vi "UHR-Fleezers Control (host) -Leonardo 04-2018 V1.vi"(0 "Tab Control":T5(tab)=enum."Trap Control (RF)") -> ()   [LabVIEW 2013] (continued)
  n85 = xnode "Read/Write Control"("FPGA VI Reference In"=w151, "error in"=w171, "ai count"="AI Count (ticks)", "Interlace ON/OFF"=w137, "Number Interlace Cycles"=w136, "Set 1"=w16, "Set 2"=w15, "Set 3"=w14, "FB On/Off Set 1"=w258, "FB On/Off Set 2"=w257, "Interlace Off Parameters"=w135, "FB Setpoint Set 1"=w249, "FB Setpoint Set 2"=w248, "FB Gains"="PID gains", "FB output range"=cluster{"output high":i16, "output low":i16} {"output high"=3000, "output low"=0} ("FB output range 1"), "Cycles per step"=w234, "Scan BD"=w246, "Number of scans"=w230, "Scan steps"=w235, "Scan freq.  increment"=w236, "AO1 (Y)"=w218, "AO2 (X)"=w217, "Scan freq.  increment (MCL)"=w211, "Scan steps (MCL)"=w210, "Cycles per step (MCL)"=w209, "Number of scans (MCL)"=w208, "MCL count"=w134, "Cont. Scan (MCL)"=w207, "MCL Scan Axis"=w201, "1D or 2D Scan?"=w154, "N of AI1 Int Acq Sets"=w191, "BD 1 Delay (ticks)"="Freq switch delay", "Amp switch delay"="Amp switch delay", "Swap F1 and F2"="Swap F1 and F2", "APD Acq Rate Count"=w159, "APD to FIFO"=FALSE, "APD Gate Operating Mode"="APD Gate", "APD Gate ON Count"="APD Gate ON Count", "APD Gate OFF Count"="APD Gate OFF Count", "Invert APD Gate"="Invert APD Gate", "DIO count 1 (ticks)"="DIO count 1 (ticks)", "DIO count 2 (ticks)"="DIO count 2 (ticks)", "DIO count 3 (ticks)"="DIO count 3 (ticks)", "APD 1 AO scale factor"="APD 1 AO Mult.", "APD 2 AO scale factor"="APD 2 AO Mult.", "Diff FB Measurement?"=w21, "Dynamic Force FB (Ronen)"=w20, "Negate Diff?"=w19, "Next trap write delay (ticks)"="Next trap write delay (ticks)", "Phase offset method"="Phase offset method", "Phase Trap 1"="Phase increment trap 1", "RF phase reset before cycles"="RF phase reset before cycles", "Phase Trap 2"="Phase increment trap 2") -> ("FPGA VI Reference Out"=w129:T20, "error out"=w131:errorcluster)  [unwired: 1 in]
  n86 = local read "Green Laser ON/Interlacing"() -> (w132:bool)
  n87 = local read "Green laser mode"() -> (w133:enum32{"Laser ON", "Laser OFF", "Interlace"})
  n88 = local read "GI Frequency, OFF count"() -> (w125:u32)
  n89 = local read "GI Frequency, ON count"() -> (w124:u32)
  n90 = Multiply(x="Current When FB OFF (%)", y=655.35) -> (x*y=w115:dbl)
  n91 = local read "Green FB Count"() -> (w123:u32)
  n92 = Multiply(x="Green FB Setpoint (mV)", y=3.2767) -> (x*y=w112:dbl)
  n93 = To Unsigned Word Integer(number=w115) -> (unsigned 16bit integer=w113:u16)
  n94 = local read "Invert GI"() -> (w127:bool)
  n95 = To Word Integer(number=w112) -> (16bit integer=w110:i16)
  n96 = case shown="True" w132 {
    tunnel: w133 -> [_ w293]
    tunnel: [enum32{"Laser ON", "Laser OFF", "Interlace"}."Laser OFF" ("Green laser mode") w293] -> w126
    frame False {
    }
    frame True {
    }
  }
  n97 = local read "Trap Pos. AI1 X Pre-scale"() -> (w81:u16)
  n98 = local read "Trap Pos FB Monitor\nT1 or T2"() -> (w88:bool)
  n99 = local read "Trap Pos FB Int Count"() -> (w78:u16)
  n100 = local read "Trap Pos FB Negate Action"() -> (w87:bool)
  n101 = local read "Trap Pos. FB Offset Factor"() -> (w86:i64)
  n102 = local read "Trap Pos. FB Mult Factor"() -> (w85:i64)
  n103 = local read "Trap Pos. FB Gains"() -> (w83:T11)
  n104 = local read "Trap Pos. FB Range"() -> (w84:T12)
  n105 = xnode "Read/Write Control"("FPGA VI Reference In"=w129, "error in"=w131, "Green interlace ON count 2"=w124, "Green interlace OFF count 2"=w125, "Invert GI 2"=w127, "Operating Mode 2"=w126, "Green FB Gains"="Green FB Gains", "Green FB Setpoint"=w110, "Green FB On/Off"="Green FB On/Off", "Current Out"=w113, "Green int current ON count adj"="Green int current ON count adj", "Green FB Count"=w123, "Operating Mode"=w126, "Green interlace OFF count"=w125, "Green interlace ON count"=w124, "Invert GI"=w127, "Trap Pos FB Monitor T1 or T2"=w88, "Trap Pos FB Negate Action"=w87, "Trap Pos. FB Offset Factor"=w86, "Trap Pos. FB Mult Factor"=w85, "Trap pos. FB Range"=w84, "Trap Pos. FB Gains"=w83, "Force feedback"=FALSE, "AI1 X Scale"=w81, "Trap Pos to FIFO"=TRUE, "Trap Pos FB Int Count"=w78) -> ("FPGA VI Reference Out"=w128:T20, "error out"=w130:errorcluster)
  n106 = xnode "Invoke Method"("FPGA VI Reference In"=w128, "error in"=w130, "Requested Depth"="Trap AI FIFO Depth") -> ("FPGA VI Reference Out"=w91:T20, "error out"=w90:errorcluster)  [unwired: 1 out]
  n107 = xnode "Invoke Method"("FPGA VI Reference In"=w91, "error in"=w90, "Requested Depth"="Trap Position FIFO Depth") -> ("FPGA VI Reference Out"=w4:T20, "error out"=w2:errorcluster)  [unwired: 1 out]
  n108 = xnode "Invoke Method"("FPGA VI Reference In"=w4, "error in"=w2, "Requested Depth"="APD FIFO Depth (requires restart)") -> ("FPGA VI Reference Out"=w3:T20, "error out"=w1:errorcluster)  [unwired: 1 out]
  n109 = flat-sequence {
    tunnel: w152 -> [w298]
    tunnel: [w298] -> w151
    tunnel: [w294] -> w37
    tunnel: [w297] -> w150
    tunnel: [w296] -> w148
    tunnel: [w295] -> w149
    frame #0 {
      w295 = T16 {"Minimum"=60.0, "Maximum"=90.0, "Increment"=1.0} ("Min Max Inc")
      w296 = T16 {"Minimum"=0.0, "Maximum"=75.0, "Increment"=1.0} ("Data Entry Limits")
      w294 = T16 {"Minimum"=60.0, "Maximum"=90.0, "Increment"=1.0} ("Min Max Inc")
      w297 = T16 {"Minimum"=0.0, "Maximum"=75.0, "Increment"=1.0} ("Data Entry Limits")
      n110 = property on="BD 2 Frequency 1 (MHz)" class="DigNum (strict)"("Data Range"=w295) -> ()  [unwired: 2 in, 2 out]
      n111 = property on="BD 2 Frequency 3 (MHz)" class="DigNum (strict)"("Data Range"=w295) -> ()  [unwired: 2 in, 2 out]
      n112 = property on="BD 2 Frequency 2 (MHz)" class="DigNum (strict)"("Data Range"=w295) -> ()  [unwired: 2 in, 2 out]
      n113 = property on="BD 1 Frequency 1 (MHz)" class="DigNum (strict)"("Data Range"=w294) -> ()  [unwired: 2 in, 2 out]
      n114 = property on="BD 1 Frequency 2 (MHz)" class="DigNum (strict)"("Data Range"=w294) -> ()  [unwired: 2 in, 2 out]
      n115 = property on="BD 1 Frequency 3 (MHz)" class="DigNum (strict)"("Data Range"=w294) -> ()  [unwired: 2 in, 2 out]
      n116 = property on="BD 2 Amplitude 1 (%)" class="DigNum (strict)"("Data Range"=w296) -> ()  [unwired: 2 in, 2 out]
      n117 = property on="BD 2 Amplitude 2 (%)" class="DigNum (strict)"("Data Range"=w296) -> ()  [unwired: 2 in, 2 out]
      n118 = property on="BD 2 Amplitude 3 (%)" class="DigNum (strict)"("Data Range"=w296) -> ()  [unwired: 2 in, 2 out]
      n119 = property on="BD 1 Amplitude 3 (%)" class="DigNum (strict)"("Data Range"=w297) -> ()  [unwired: 2 in, 2 out]
      n120 = property on="BD 1 Amplitude 2 (%)" class="DigNum (strict)"("Data Range"=w297) -> ()  [unwired: 2 in, 2 out]
      n121 = property on="BD 1 Amplitude 1 (%)" class="DigNum (strict)"("Data Range"=w297) -> ()  [unwired: 2 in, 2 out]
      "X RF Frequency Limits (MHz)" <- w294
      "X RF Amplitude Limits (%)" <- w297
      "Y RF Amplitude Limits (%)" <- w296
      "Y RF Frequency Limits (MHz)" <- w295
    }
  }
  n122 = xnode "Invoke Method"("FPGA VI Reference In"=w3, "error in"=w1) -> ("FPGA VI Reference Out"=w57:T20, "error out"=w56:errorcluster)  [unwired: 1 in]
  n123 = flat-sequence "Initial FPGA Loop Relative Phase Adjustment" {
    tunnel: "Initial Phase Adjustment (APD 2 Gate)" -> [w300]
    tunnel: "Initial Phase Adjustment (GI) 2" -> [w301]
    tunnel: "Initial Phase Adj. (MCL)" -> [w302]
    tunnel: w56 -> [w303]
    tunnel: w57 -> [w304]
    tunnel: "Initial Phase Adjustment (GI)" -> [w305]
    tunnel: "Initial Phase Adjustment (AI1)" -> [w306]
    tunnel: [w306] -> w66
    tunnel: [w305] -> w65
    tunnel: [w304] -> w64
    tunnel: [w303] -> w63
    tunnel: [w302] -> w62
    tunnel: [w301] -> w61
    tunnel: [w300] -> w60
    tunnel: [w318] -> w177
    tunnel: [w312] -> w175
    tunnel: "Initial Phase Adjustment (APD Acq)" -> [w311]
    tunnel: "Initial Phase Adjustment (APD 1 Gate)" -> [w310]
    tunnel: "Initial Phase Adjustment (Green FB)" -> [w309]
    tunnel: w66 -> [w317]
    tunnel: w65 -> [w316]
    tunnel: w64 -> [w315]
    tunnel: w63 -> [w314]
    tunnel: w62 -> [w313]
    tunnel: w61 -> [w308]
    tunnel: w60 -> [w307]
    tunnel: w177 -> [w320]
    tunnel: [w321] -> w176
    tunnel: w175 -> [w321]
    tunnel: [w320] -> w174
    tunnel: w176 -> [w324]
    tunnel: w174 -> [w323]
    tunnel: [w326] -> w173
    tunnel: [w325] -> w172
    tunnel: [w328] -> w55
    tunnel: [w329] -> w58
    tunnel: w173 -> [w329]
    tunnel: w172 -> [w328]
    frame #0 {
      n124 = Wait (ms)(milliseconds to wait=u32 1000) -> ()  [unwired: 1 out]
    }
    frame #1 {
      n125 = xnode "Read/Write Control"("FPGA VI Reference In"=w315, "error in"=w314, "Phase count adjustment"=w317, "Phase count adjustment (GI)"=w316, "Phase count adjustment (MCL)"=w313, "Phase Count Adjustment (APD Acq)"=w311, "Phase count adjustment (APD 1 Gate)"=w310, "Phase count adjustment (APD 2 Gate)"=w307, "Phase count adjustment (Green FB)"=w309, "Phase count adjustment (GI) 2"=w308) -> ("FPGA VI Reference Out"=w312:T20, "error out"=w318:errorcluster)
    }
    frame #2 {
      n126 = Wait (ms)(milliseconds to wait=u32 1000) -> ()  [unwired: 1 out]
    }
    frame #3 {
      w322 = TRUE
      n127 = xnode "Read/Write Control"("FPGA VI Reference In"=w324, "error in"=w323, "+ phase"=w322, "+ phase (GI)"=w322, "+ phase (MCL)"=w322, "+ phase (APD Acq)"=w322, "+ phase (APD 1 Gate)"=w322, "+ phase (APD 2 Gate)"=w322, "+ phase (Green FB)"=w322, "+ phase (GI) 2"=w322) -> ("FPGA VI Reference Out"=w325:T20, "error out"=w326:errorcluster)
    }
    frame #4 {
      n128 = Wait (ms)(milliseconds to wait=u32 1000) -> ()  [unwired: 1 out]
    }
  }
  n129 = Unbundle By Name(w37) -> ("Minimum"=w36:dbl, "Maximum"=w35:dbl)
  n130 = local read "Phase adj. (Green FB)"() -> (w146:i16)
  n131 = local read "Phase adj. (GI) 2"() -> (w116:i16)
  n132 = local read "Phase adjust (MCL)"() -> (w202:i16)
  n133 = local read "Phase adj. (AI1)"() -> (w204:i16)
  n134 = local read "Phase adj. (GI)"() -> (w203:i16)
  n135 = Multiply(x=w36, y=w34) -> (x*y=w32:dbl)
  n136 = Multiply(x=w35, y=w34) -> (x*y=w33:dbl)
  n137 = Multiply(x=49152000.0, y=6.0) -> (x*y=w26:dbl)
  n138 = Scale By Power Of 2(n=w31, x=w32) -> (x*2^n=w28:dbl)
  n139 = Scale By Power Of 2(n=w31, x=w33) -> (x*2^n=w27:dbl)
  n140 = xnode "Read/Write Control"("FPGA VI Reference In"=w55, "error in"=w58, "Phase count adjustment"=w204, "Phase count adjustment (GI)"=w203, "Phase count adjustment (MCL)"=w202, "Phase Count Adjustment (APD Acq)"="Phase Adj. (APD Acq)", "Phase count adjustment (APD 1 Gate)"="Phase Adj. (APD 1 Gate)", "Phase count adjustment (APD 2 Gate)"="Phase Adj. (APD 2 Gate)", "Phase count adjustment (Green FB)"=w146, "Phase count adjustment (GI) 2"=w116) -> ("FPGA VI Reference Out"=w12:T20, "error out"=w11:errorcluster)
  n141 = Divide(x=w27, y=w26) -> (x/y=w24:dbl)
  n142 = Divide(x=w28, y=w26) -> (x/y=w25:dbl)
  n143 = To Unsigned Quad Integer(1:w25) -> (0:w23:u64)
  n144 = To Unsigned Quad Integer(1:w24) -> (0:w22:u64)
  n145 = xnode "Read/Write Control"("FPGA VI Reference In"=w12, "FB Min frequency"=w23, "FB Max Frequency"=w22) -> ()  [unwired: 1 in, 2 out]
  n146 = call "set RF board frequency - interlace.vi"("Board 2 Frequency Limits"=w149, "Board 1 Frequency Limits"=w37, "error in"=w11, "FPGA VI Reference In"=w12, "Board 2 Frequency 3 (MHz)"="BD 2 Frequency 3 (MHz)", "Board 1 Frequency 3 (MHz)"="BD 1 Frequency 3 (MHz)", "Board 2 Frequency 2 (MHz)"="BD 2 Frequency 2 (MHz)", "Board 2 Frequency 1 (MHz)"="BD 2 Frequency 1 (MHz)", "Board 1 Frequency 2 (MHz)"="BD 1 Frequency 2 (MHz)", "Board 1 Frequency 1  (MHz)"="BD 1 Frequency 1 (MHz)") -> ("error out"=w269:errorcluster, "FPGA VI Reference Out"=w270:T20)
  n147 = call "set RF board amplitude - interlace.vi"("Board 2 Amplitude Limits"=w148, "Board 1 Amplitude Limits"=w150, "error in"=w269, "FPGA VI Reference In"=w270, "Board 2 Amplitude 3 (%)"="BD 2 Amplitude 3 (%)", "Board 1 Amplitude 3 (%)"="BD 1 Amplitude 3 (%)", "Board 2 Amplitude 2 (%)"="BD 2 Amplitude 2 (%)", "Board 2 Amplitude 1 (%)"="BD 2 Amplitude 1 (%)", "Board 1 Amplitude 2 (%)"="BD 1 Amplitude 2 (%)", "Board 1 Amplitude 1 (%)"="BD 1 Amplitude 1 (%)") -> ("error out"=w53:errorcluster, "FPGA VI Reference Out"=w54:T20)
  n148 = flat-sequence {
    tunnel: w54 -> [w331]
    tunnel: w53 -> [w330]
    tunnel: [w331] -> w262
    tunnel: [w330] -> w261
    tunnel: [w339] -> w260
    tunnel: w262 -> [w339]
    tunnel: [w338] -> w259
    tunnel: w261 -> [w338]
    tunnel: w260 -> [w342]
    tunnel: w259 -> [w341]
    tunnel: [w342] -> w49
    tunnel: [w341] -> w48
    tunnel: [w348] -> w75
    tunnel: [w352] -> w59
    tunnel: w49 -> [w352]
    tunnel: w48 -> [w347]
    frame #0 {
      n149 = local read "Trap 1 (ON/OFF)"() -> (w332:bool)
      n150 = local write "Saving..."(FALSE ("Saving Data")) -> ()
      n151 = local write "Stop All"(FALSE ("Stop All")) -> ()
      n152 = local write "Index"(1.0 ("Index")) -> ()
      n153 = property on="Trap 1 ON" class="Bool (strict)"("Value"=w332) -> ()  [unwired: 2 in, 2 out]
      "Manipulating Trap" <- FALSE ("Manipulating Trap")
    }
    frame #1 {
      n154 = local read "Trap 2 (ON/OFF)"() -> (w337:bool)
      n155 = Wait (ms)(milliseconds to wait=u32 50) -> ()  [unwired: 1 out]
      n156 = property on="Trap 2 ON" class="Bool (strict)"("Val(Sgnl)"=w337) -> ()  [unwired: 2 in, 2 out]
    }
    frame #2 {
      n157 = local read "Scan Range (nm)"() -> (w343:dbl)
      n158 = call "Update messages.vi"("Message to add"="UHR-Fleezers ready.", "Old message string"="") -> ("New message string"=w346:string)
      n159 = local write "Messages"(w346) -> ()
      n160 = property on="Scan Range (nm)" class="DigNum (strict)"("Val(Sgnl)"=w343) -> ()  [unwired: 2 in, 2 out]
    }
    frame #3 {
      n161 = call "hamilton_controller.vi"("error in"=w347, "action"=T21."CONNECT") -> ("error out"=w349:errorcluster)  [unwired: 9 in]
      n162 = call "hamilton_controller.vi"("error in"=w349, "action"=T21."INITIALIZE VALVES") -> ("error out"=w348:errorcluster)  [unwired: 9 in]
    }
  }
  n163 = Subtract(x="BD 1 Frequency 1 (MHz)", y="BD 1 Frequency 2 (MHz)") -> (x-y=w190:dbl)
  n164 = Subtract(x="BD 2 Frequency 1 (MHz)", y="BD 2 Frequency 2 (MHz)") -> (x-y=w189:dbl)
  n165 = Square(x=w189) -> (x^2=w187:dbl)
  n166 = Square(x=w190) -> (x^2=w188:dbl)
  n167 = Add(x=w188, y=w187) -> (x+y=w186:dbl)
  n168 = Square Root(x=w186) -> (sqrt(x)=w185:dbl)
  n169 = local write "Trap Delta (MHz)"(w185) -> ()
  n170 = call "IMAQ Create"("Image Name"="APD 1 Image", "Image Type"=w97) -> ("New Image"=w96:T3)  [unwired: 3 in, 1 out]
  n171 = call "IMAQ Create"("Image Name"="APD 2 Image", "Image Type"=w97) -> ("New Image"=w95:T3)  [unwired: 3 in, 1 out]
  n172 = call "IMAQ Create"("Image Name"="Det. X Image", "Image Type"=w97) -> ("New Image"=w94:T3)  [unwired: 3 in, 1 out]
  n173 = call "IMAQ Create"("Image Name"="Det. Y Image", "Image Type"=w97) -> ("New Image"=w93:T3)  [unwired: 3 in, 1 out]
  n174 = Bundle("New Image"=w96, "New Image"=w95, "New Image"=w94, "New Image"=w93) -> (w92:T22)  [unwired: 1 in]
  n175 = Current VI's Path() -> (path=w38:path)
  n176 = Concatenate Strings("N.D.", "\r\n") -> (w42:string)
  n177 = Strip Path(path=w38) -> (stripped path=w39:path)  [unwired: 1 out]
  n178 = Initialize Array(w42, 4, 3) -> (w45:string[][])
  n179 = Build Path(base path=w39, name or relative path="Locations.txt") -> (appended path=→"Location path":path)
  n180 = local write "Location Matrix"(w45) -> ()
  n181 = while {
    stop <- w353 stop-if-true
    n182 = event shown="[6] \"VISA Clear\": Value Change" {
      selector: _ -> [_ _ _ _ _ _ _ _ _]
      dyn-events: _ -> [_ _ _ _ _ _ _ _ _]
      timeout: 10 -> [_ _ _ _ _ _ _ _ _]
      tunnel: [FALSE _ _ _ _ _ _ _ TRUE] -> w353
      event Timeout {
        # "Change the trajectory mode to Jog"
        # "Query and display stage positions"
        # "Setting ESP300 left and right limits for Z-axis, input in mm"
        # "Display Selected Location"
        n183 = event-data() -> ()  [unwired: 1 in, 2 out]
        n184 = local read "Capture Locations"() -> (w378:i32)
        n185 = local read "Location Matrix"() -> (w379:string[][])
        n186 = Concatenate Strings("1TP;\n2TP;\n3TP;\n1MD?;\n2MD?;\n3MD?" ("Substring"), "\r") -> (w362:string)
        n187 = local read "ESP Port"() -> (w365:refnum<visa-resource-name>)
        n188 = Index Array(array=w379, index (row)=w378) -> (element=w377:string[])  [unwired: 1 in]
        n189 = local read "ESP Port"() -> (w374:refnum<visa-resource-name>)
        n190 = VISA Write(VISA resource name=w365, write buffer=w362, error in (no error)="error in") -> (VISA resource name out=w363:refnum<visa-resource-name>, error out=w361:errorcluster)  [unwired: 1 out]
        n191 = Concatenate Strings("3SL" ("Substring"), "ESP ZL-Limit", ";3SR", "ESP ZR-Limit", "\r") -> (w373:string)
        n192 = Array To Cluster(array=w377) -> (cluster=w376:T23)
        n193 = case shown="True" TRUE ("Case Constant\n(See Context Help)") {
          tunnel: w363 -> [_ w417]
          tunnel: w361 -> [w398 w416]
          tunnel: [w398 w400] -> w367
          frame False {
          }
          frame True {
            w410 = u16 10 items=["1.0"=10, "1.5"=15, "2.0"=20] ("Serial Settings:Stop Bits")
            w411 = u16 0 items=["None", "Odd", "Even", "Mark", "Space"] ("Serial Settings:Parity")
            n194 = property class="Instr"(reference=w417, error in=w416, "Baud"=u32 921600 ("Serial Settings:Baud Rate"), "Data Bits"=u16 8 ("Serial Settings:Data Bits"), "Parity"=w411, "Stop Bits"=w410) -> (reference out=w415:refnum<visa-resource-name>, error out=w414:errorcluster, "Bytes at Port"=w399:u32)
            n195 = Wait (ms)(milliseconds to wait=u32 10) -> ()  [unwired: 1 out]
            n196 = VISA Read(VISA resource name=w415, byte count=w399, error in (no error)=w414) -> (VISA resource name out=w423:refnum<visa-resource-name>, read buffer=→"X Pos":string, error out=w424:errorcluster)  [unwired: 1 out]
            n197 = VISA Read(VISA resource name=w423, byte count=w399, error in (no error)=w424) -> (VISA resource name out=w421:refnum<visa-resource-name>, read buffer=→"Y Pos":string, error out=w422:errorcluster)  [unwired: 1 out]
            n198 = VISA Read(VISA resource name=w421, byte count=w399, error in (no error)=w422) -> (VISA resource name out=w409:refnum<visa-resource-name>, read buffer=→"Z Pos Pos":string, error out=w408:errorcluster)  [unwired: 1 out]
            n199 = VISA Read(VISA resource name=w409, byte count=w399, error in (no error)=w408) -> (VISA resource name out=w405:refnum<visa-resource-name>, read buffer=→"X Motion":string, error out=w406:errorcluster)  [unwired: 1 out]
            n200 = VISA Read(VISA resource name=w405, byte count=w399, error in (no error)=w406) -> (VISA resource name out=w404:refnum<visa-resource-name>, read buffer=→"Y Motion":string, error out=w402:errorcluster)  [unwired: 1 out]
            n201 = VISA Read(VISA resource name=w404, byte count=w399, error in (no error)=w402) -> (read buffer=→"Z motion":string, error out=w400:errorcluster)  [unwired: 2 out]
          }
        }
        "error out" <- w367
        n202 = VISA Write(VISA resource name=w374, write buffer=w373) -> ()  [unwired: 1 in, 3 out]
        n203 = local write item#483(w376) -> ()
        n204 = disable-structure shown="Disabled" {
          frame Disabled {
            # "Change Low Jog Velocity"
            # "Change High Jog Velocity"
            n205 = Concatenate Strings("1JH" ("Substring"), "Axis 1", "2JH" ("Substring"), "Axis 2", "3JH" ("Substring"), "Axis 3", "\r") -> (w397:string)
            n206 = local read "ESP Port"() -> (w396:refnum<visa-resource-name>)
            n207 = VISA Write(VISA resource name=w396, write buffer=w397) -> ()  [unwired: 1 in, 3 out]
            n208 = Concatenate Strings("1JW" ("Substring"), "Axis 1", "2JW" ("Substring"), "Axis 2", "3JW" ("Substring"), "Axis 3", "\r") -> (w388:string)
            n209 = local read "ESP Port"() -> (w387:refnum<visa-resource-name>)
            n210 = VISA Write(VISA resource name=w387, write buffer=w388) -> ()  [unwired: 1 in, 3 out]
          }
          frame Enabled {
          }
        }
        n211 = local read "ESP Port"() -> (w355:refnum<visa-resource-name>)
        n212 = Concatenate Strings("1TJ3;\n2TJ3;\n3TJ3" ("Substring"), "\r") -> (w356:string)
        n213 = VISA Write(VISA resource name=w355, write buffer=w356) -> ()  [unwired: 1 in, 3 out]
      }
      event "Goto Top (F6)": Value Change {
        n214 = event-data() -> ()  [unwired: 1 in, 5 out]
        n215 = stacked-sequence {
          frame #0 {
            # "stop motions of all axes before going to avoid reversing of direction"
            n216 = local read "ESP Port"() -> (w429:refnum<visa-resource-name>)
            n217 = Concatenate Strings("ST" ("Substring"), "\r") -> (w426:string)
            n218 = VISA Write(VISA resource name=w429, write buffer=w426) -> ()  [unwired: 1 in, 3 out]
          }
          frame #1 {
            n219 = Wait (ms)(milliseconds to wait=u32 50) -> ()  [unwired: 1 out]
          }
          frame #2 {
            # "Change the trajectory mode to Trapezoidal"
            n220 = local read "ESP Port"() -> (w434:refnum<visa-resource-name>)
            n221 = Concatenate Strings("1TJ1;\n2TJ1;\n3TJ1" ("Substring"), "\r") -> (w431:string)
            n222 = VISA Write(VISA resource name=w434, write buffer=w431) -> ()  [unwired: 1 in, 3 out]
          }
          frame #3 {
            # "Go to Top Dispensor"
            n223 = local read "Location Matrix"() -> (w446:string[][])
            n224 = Index Array(array=w446, index (row)=0) -> (element=w442:string[])  [unwired: 1 in]
            n225 = Decimate 1D Array(w442) -> (w440:string[], w438:string[], w436:string[])
            n226 = local read "ESP Port"() -> (w443:refnum<visa-resource-name>)
            n227 = Concatenate Strings("1PA" ("Substring"), w440, "2PA" ("Substring"), w438, "3PA" ("Substring"), w436, "\r") -> (w444:string)
            n228 = VISA Write(VISA resource name=w443, write buffer=w444) -> ()  [unwired: 1 in, 3 out]
          }
          frame #4 {
            n229 = Wait (ms)(milliseconds to wait=u32 100) -> ()  [unwired: 1 out]
          }
          frame #5 {
            # "Change the trajectory mode to Jog"
            n230 = local read "ESP Port"() -> (w451:refnum<visa-resource-name>)
            n231 = Concatenate Strings("1TJ3;\n2TJ3;\n3TJ3" ("Substring"), "\r") -> (w448:string)
            n232 = VISA Write(VISA resource name=w451, write buffer=w448) -> ()  [unwired: 1 in, 3 out]
          }
        }
      }
      event "Goto Exp (F8)": Value Change {
        n233 = event-data() -> ()  [unwired: 1 in, 5 out]
        n234 = stacked-sequence {
          frame #0 {
            # "stop motions of all axes before going to avoid reversing of direction"
            n235 = local read "ESP Port"() -> (w455:refnum<visa-resource-name>)
            n236 = Concatenate Strings("ST" ("Substring"), "\r") -> (w452:string)
            n237 = VISA Write(VISA resource name=w455, write buffer=w452) -> ()  [unwired: 1 in, 3 out]
          }
          frame #1 {
            n238 = Wait (ms)(milliseconds to wait=u32 50) -> ()  [unwired: 1 out]
          }
          frame #2 {
            # "Change the trajectory mode to Trapezoidal"
            n239 = local read "ESP Port"() -> (w460:refnum<visa-resource-name>)
            n240 = Concatenate Strings("1TJ1;\n2TJ1;\n3TJ1" ("Substring"), "\r") -> (w457:string)
            n241 = VISA Write(VISA resource name=w460, write buffer=w457) -> ()  [unwired: 1 in, 3 out]
          }
          frame #3 {
            # "Go to Experimental"
            n242 = local read "Location Matrix"() -> (w472:string[][])
            n243 = Index Array(array=w472, index (row)=2) -> (element=w468:string[])  [unwired: 1 in]
            n244 = Decimate 1D Array(w468) -> (w466:string[], w464:string[], w462:string[])
            n245 = Concatenate Strings("1PA" ("Substring"), w466, "2PA" ("Substring"), w464, "3PA" ("Substring"), w462, "\r") -> (w470:string)
            n246 = local read "ESP Port"() -> (w469:refnum<visa-resource-name>)
            n247 = VISA Write(VISA resource name=w469, write buffer=w470) -> ()  [unwired: 1 in, 3 out]
          }
          frame #4 {
            n248 = Wait (ms)(milliseconds to wait=u32 200) -> ()  [unwired: 1 out]
          }
          frame #5 {
            # "Change the trajectory mode to Jog"
            n249 = local read "ESP Port"() -> (w474:refnum<visa-resource-name>)
            n250 = Concatenate Strings("1TJ3;\n2TJ3;\n3TJ3" ("Substring"), "\r") -> (w477:string)
            n251 = VISA Write(VISA resource name=w474, write buffer=w477) -> ()  [unwired: 1 in, 3 out]
          }
        }
      }
      event "Goto Bottom (F7)": Value Change {
        n252 = event-data() -> ()  [unwired: 1 in, 5 out]
        n253 = stacked-sequence {
          frame #0 {
            # "stop motions of all axes before going to avoid reversing of direction"
            n254 = local read "ESP Port"() -> (w481:refnum<visa-resource-name>)
            n255 = Concatenate Strings("ST" ("Substring"), "\r") -> (w478:string)
            n256 = VISA Write(VISA resource name=w481, write buffer=w478) -> ()  [unwired: 1 in, 3 out]
          }
          frame #1 {
            n257 = Wait (ms)(milliseconds to wait=u32 50) -> ()  [unwired: 1 out]
          }
          frame #2 {
            # "Change the trajectory mode to Trapezoidal"
            n258 = local read "ESP Port"() -> (w486:refnum<visa-resource-name>)
            n259 = Concatenate Strings("1TJ1;\n2TJ1;\n3TJ1" ("Substring"), "\r") -> (w483:string)
            n260 = VISA Write(VISA resource name=w486, write buffer=w483) -> ()  [unwired: 1 in, 3 out]
          }
          frame #3 {
            # "Go to Bottom Dispensor"
            n261 = local read "Location Matrix"() -> (w498:string[][])
            n262 = Index Array(array=w498, index (row)=1) -> (element=w494:string[])  [unwired: 1 in]
            n263 = Decimate 1D Array(w494) -> (w492:string[], w490:string[], w488:string[])
            n264 = Concatenate Strings("1PA" ("Substring"), w492, "2PA" ("Substring"), w490, "3PA" ("Substring"), w488, "\r") -> (w496:string)
            n265 = local read "ESP Port"() -> (w495:refnum<visa-resource-name>)
            n266 = VISA Write(VISA resource name=w495, write buffer=w496) -> ()  [unwired: 1 in, 3 out]
          }
          frame #4 {
            n267 = Wait (ms)(milliseconds to wait=u32 200) -> ()  [unwired: 1 out]
          }
          frame #5 {
            # "Change the trajectory mode to Jog"
            n268 = local read "ESP Port"() -> (w500:refnum<visa-resource-name>)
            n269 = Concatenate Strings("1TJ3;\n2TJ3;\n3TJ3" ("Substring"), "\r") -> (w503:string)
            n270 = VISA Write(VISA resource name=w500, write buffer=w503) -> ()  [unwired: 1 in, 3 out]
          }
        }
      }
      event "Capture": Value Change {
        n271 = event-data() -> ()  [unwired: 1 in, 5 out]
        n272 = local read "Capture Locations"() -> (w504:i32)
        n273 = local read "Z Pos Pos"() -> (w505:string)
        n274 = local read "X Pos"() -> (w507:string)
        n275 = local read "Y Pos"() -> (w506:string)
        n276 = case shown="1" w504 {
          selector: w504 -> [w511 w518 w525 w532]
          tunnel: w507 -> [w514 w521 w528 w535]
          tunnel: w506 -> [w513 w520 w527 w534]
          tunnel: w505 -> [w512 w519 w526 w533]
          frame 0, Default {
            # "Capture Top Dispensor Location"
            n277 = local read "Location Matrix"() -> (w510:string[][])
            n278 = Build Array(w514, w513, w512) -> (w509:string[])
            n279 = Replace Array Subset(array=w510, new element=w509, index (row)=w511) -> (w508:string[][])  [unwired: 1 in]
            n280 = local write "Location Matrix"(w508) -> ()
          }
          frame 1 {
            # "Capture Bottom Dispensor Location"
            n281 = local read "Location Matrix"() -> (w517:string[][])
            n282 = Build Array(w521, w520, w519) -> (w516:string[])
            n283 = Replace Array Subset(array=w517, new element=w516, index (row)=w518) -> (w515:string[][])  [unwired: 1 in]
            n284 = local write "Location Matrix"(w515) -> ()
          }
          frame 2 {
            # "Capture Experimental Region Location"
            n285 = local read "Location Matrix"() -> (w524:string[][])
            n286 = Build Array(w528, w527, w526) -> (w523:string[])
            n287 = Replace Array Subset(array=w524, new element=w523, index (row)=w525) -> (w522:string[][])  [unwired: 1 in]
            n288 = local write "Location Matrix"(w522) -> ()
          }
          frame 3 {
            # "Capture Other Location"
            n289 = local read "Location Matrix"() -> (w531:string[][])
            n290 = Build Array(w535, w534, w533) -> (w530:string[])
            n291 = Replace Array Subset(array=w531, new element=w530, index (row)=w532) -> (w529:string[][])  [unwired: 1 in]
            n292 = local write "Location Matrix"(w529) -> ()
          }
        }
      }
      event "Save": Value Change {
        # "reshape Location Matrix to 1-D array to write"
        n293 = event-data() -> ()  [unwired: 1 in, 5 out]
        n294 = local read "Location Matrix"() -> (w539:string[][])
        n295 = local read "Location path"() -> (w536:path)
        n296 = Reshape Array(w539, 12) -> (w537:string[])
        n297 = Write to Text File(file (use dialog)=w536, text=w537) -> ()  [unwired: 2 in, 3 out]
      }
      event "VISA Clear": Value Change {
        n298 = event-data() -> ()  [unwired: 1 in, 5 out]
        n299 = local read "ESP Port"() -> (w540:refnum<visa-resource-name>)
        n300 = VISA Clear(VISA resource name=w540) -> ()  [unwired: 1 in, 2 out]
      }
      event "Activate Joystick": Value Change {
        # "Change the trajectory mode to Jog"
        n301 = event-data() -> ()  [unwired: 1 in, 5 out]
        n302 = disable-structure shown="Disabled" {
          frame Disabled {
            n303 = case shown="True" "Activate Joystick" {
              frame False {
              }
              frame True {
                # "Change the trajectory mode to Jog"
                n304 = local read "ESP Port"() -> (w549:refnum<visa-resource-name>)
                n305 = Concatenate Strings("1TJ3;\n2TJ3;\n3TJ3" ("Substring"), "\r") -> (w546:string)
                n306 = VISA Write(VISA resource name=w549, write buffer=w546) -> ()  [unwired: 1 in, 3 out]
              }
            }
          }
          frame Enabled {
          }
        }
        n307 = local read "ESP Port"() -> (w541:refnum<visa-resource-name>)
        n308 = Concatenate Strings("1TJ3;\n2TJ3;\n3TJ3" ("Substring"), "\r") -> (w544:string)
        n309 = VISA Write(VISA resource name=w541, write buffer=w544) -> ()  [unwired: 1 in, 3 out]
      }
      event "Stop All": Mouse Down {
        n310 = event-data() -> ()  [unwired: 1 in, 5 out]
      }
    }
  }
  n311 = disable-structure shown="Disabled" {
    disable-tunnel: w59 -> [w579 _]
    frame Disabled {
      w574 = T17 0 items=["Grayscale (U8)", "Grayscale (I16)", "Grayscale (SGL)", "Complex (CSG)", "RGB (U32)", "HSL (U32)", "RGB (U64)", "Grayscale (U16)"] ("Image Type")
      n312 = call <vilib>:"IMAQ Init.vi"("Interface Name"="img0") -> ("error out"=w576:errorcluster, "IMAQ Session Out"=w578:refnum<k11>)  [unwired: 9 in]
      n313 = call <vilib>:"IMAQ Grab Setup.vi"("error in (no error)"=w576, "IMAQ Session In"=w578) -> ("error out"=w572:errorcluster, "IMAQ Session Out"=w573:refnum<k11>)  [unwired: 8 in]
      n314 = call "IMAQ Create"("Image Name"="untitled", "Image Type"=w574) -> ("New Image"=w571:T3)  [unwired: 3 in, 1 out]
      n315 = call <vilib>:"Application Directory.vi"() -> ("Application Directory"=w558:path)
      n316 = Build Path(base path=w558, name or relative path="_trap_screen_positions") -> (appended path=w566:path)
      n317 = Open/Create/Replace File(file path (use dialog)=w566, operation (0:open)=T24."open or create", access (0:read/write)=enum16{"read/write", "read-only", "write-only"}."read/write") -> (refnum out=w568:refnum<file>)  [unwired: 3 in, 2 out]
      n318 = local read "Trap Sets"() -> (w560:u32)
      n319 = for "Load trap positions on video screen from file." {
        N: w560 -> [_]
        tunnel: [w586] -> w561
        tunnel: w568 -> [w585]
        tunnel: [w582] -> w557 mode=indexing
        w584 = 4
        n320 = for {
          N: w584 -> [_]
          tunnel: [w590] -> w586
          tunnel: w585 -> [w589]
          tunnel: w584 -> [w588]
          tunnel: [w587] -> w583 mode=indexing
          n321 = Read from Binary File(5:w588, 11:w589) -> (2:w587:i32, 3:w590:refnum<file>)  [unwired: 4 in, 2 out]
        }
        n322 = Array To Cluster(array=w583) -> (cluster=w582:T28)
      }
      n323 = node-c288() -> (w581:T25)  [unwired: 4 in]
      n324 = timed-loop "acquire video and stage position" {
        timing: w581 -> [_]
        timing-out: [_] -> w580
        tunnel: w573 -> [w609]
        tunnel: w572 -> [w608]
        tunnel: w571 -> [w607]
        tunnel: [w606] -> w553
        tunnel: [w603] -> w554
        tunnel: [w604] -> w552
        tunnel: w579 -> [_]
        shift-right: [w600] -> w570
        shift-left: w557 -> [w601]
        tunnel: w560 -> [w598]
        stop <- w605 stop-if-true
        n325 = node-c288() -> ()  [unwired: 1 in, 1 out]
        n326 = event shown="[0] Timeout" {
          selector: _ -> [_ _ _ _]
          dyn-events: _ -> [_ _ _ _]
          timeout: 10 -> [_ _ _ _]
          tunnel: w609 -> [w620 w635 w644 w663]
          tunnel: w608 -> [w619 w637 w642 w665]
          tunnel: w607 -> [w618 w636 w643 w664]
          tunnel: [w617 w635 w644 w663] -> w606
          tunnel: [w610 w639 FALSE FALSE] -> w605
          tunnel: [w614 w637 w642 w665] -> w604
          tunnel: [w613 w636 w643 w664] -> w603
          tunnel: "radius" -> [_ _ w649 _]
          tunnel: w601 -> [w611 w638 w647 _]
          tunnel: [w611 w638 w648 cluster{i32, i32, i32, i32}[] []] -> w600
          tunnel: w598 -> [_ _ w640 _]
          event Timeout {
            n327 = event-data() -> ()  [unwired: 1 in, 2 out]
            n328 = call <vilib>:"IMAQ Grab Acquire.vi"("error in (no error)"=w619, "Image In"=w618, "IMAQ Session In"=w620) -> ("error out"=w615:errorcluster, "Image Out"=w616:T3, "IMAQ Session Out"=w617:refnum<k11>)  [unwired: 5 in, 1 out]
            n329 = case shown="True" "trap\nmarkers?" {
              tunnel: w611 -> [_ w628]
              tunnel: w616 -> [w622 w627]
              tunnel: w615 -> [w621 w626]
              tunnel: [w621 w625] -> w614
              tunnel: [w622 w623] -> w613
              frame False {
              }
              frame True {
                n330 = for {
                  tunnel: w628 -> [w634] mode=indexing
                  shift-right: [w632] -> w623
                  shift-left: w627 -> [w633]
                  tunnel: w626 -> [w631]
                  tunnel: [w630] -> w625
                  tunnel: u32 16711680 ("Color") -> [w629]
                  n331 = call "IMAQ Overlay Oval"("Color"=w629, "error in (no error)"=w631, "Bounding Rectangle"=w634, "Image"=w633) -> ("error out"=w630:errorcluster, "Image Out"=w632:T3)  [unwired: 6 in]
                }
              }
            }
            "Primary Video Display" <- w613
            n332 = Unbundle By Name(w615) -> ("status"=w610:bool)
          }
          event "Stop All": Value Change {
            n333 = event-data() -> ()  [unwired: 1 in, 5 out]
            n334 = local read "Stop All"() -> (w639:bool)
          }
          event "Primary Video Display": Mouse Down {
            n335 = event-data() -> ()  [unwired: 1 in, 7 out]
            n336 = Array Size(array=w647) -> (size(s)=w646:i32)
            n337 = Less?(x=w646, y=w640) -> (x < y?=w645:bool)
            n338 = case shown="True" w645 {
              tunnel: w649 -> [_ w659]
              tunnel: w647 -> [w650 w653]
              tunnel: [w650 w652] -> w648
              frame False {
              }
              frame True {
                n339 = property on="Primary Video Display" class="ImageControl"() -> ("Last Mouse Position"=w651:cluster{"X":i32, "Y":i32})  [unwired: 2 in, 2 out]
                n340 = Unbundle By Name(w651) -> ("X"=w661:i32, "Y"=w660:i32)
                n341 = Add(x=w660, y=w659) -> (x+y=w657:i32)
                n342 = Subtract(x=w660, y=w659) -> (x-y=w655:i32)
                n343 = Add(x=w661, y=w659) -> (x+y=w656:i32)
                n344 = Subtract(x=w661, y=w659) -> (x-y=w658:i32)
                n345 = Bundle(w658, w657, w656, w655) -> (w654:cluster{i32, i32, i32, i32})  [unwired: 1 in]
                n346 = Build Array (concatenate)(w653, w654) -> (w652:T29)
              }
            }
          }
          event "clear markers": Value Change {
            n347 = event-data() -> ()  [unwired: 1 in, 5 out]
          }
        }
        n348 = node-c288() -> ()  [unwired: 1 in, 1 out]
      }
      n349 = node-c288(w580) -> ()  [unwired: 1 out]
      n350 = Set File Position(offset (in bytes) (0)=i64 0, refnum=w561, from (0:start)=enum16{"start", "end", "current"}."start") -> (refnum out=w562:refnum<file>)  [unwired: 1 in, 1 out]
      n351 = for "Write trap positions to file so they can be remembered\nwhen program is removed from memory" {
        tunnel: w570 -> [w594] mode=indexing
        tunnel: [w592] -> w569
        tunnel: w562 -> [w591]
        n352 = Cluster To Array(cluster=w594) -> (array=w593:i32[])
        n353 = for {
          tunnel: w593 -> [w597] mode=indexing
          tunnel: [w596] -> w592
          tunnel: w591 -> [w595]
          n354 = Write to Binary File(file (use dialog)=w595, data=w597) -> (refnum out=w596:refnum<file>)  [unwired: 4 in, 2 out]
        }
      }
      n355 = Close File(refnum=w569) -> ()  [unwired: 1 in, 2 out]
      n356 = call "IMAQ Dispose"("Image"=w554, "error in (no error)"=w552) -> ("error out"=w551:errorcluster)  [unwired: 4 in]
      n357 = call <vilib>:"IMAQ Stop.vi"("error in (no error)"=w551, "IMAQ Session In"=w553) -> ("error out"=w555:errorcluster, "IMAQ Session Out"=w556:refnum<k11>)  [unwired: 8 in]
      n358 = call <vilib>:"IMAQ Close.vi"("error in (no error)"=w555, "IMAQ Session In"=w556) -> ()  [unwired: 9 in, 1 out]
    }
    frame Enabled {
    }
  }
  n359 = disable-structure shown="Enabled" {
    disable-tunnel: [w672 _] -> w70
    disable-tunnel: w59 -> [w671 _]
    frame Enabled {
      n360 = node-c288() -> (w674:T25)  [unwired: 4 out]
      n361 = timed-loop "Rough control of MCL mirror stage (debugging)" {
        tunnel: w671 -> [w677]
        tunnel: [w676] -> w672
        timing: w674 -> [_]
        timing-out: [_] -> w673
        stop <- w676 stop-if-true
        n362 = node-c288() -> ()  [unwired: 2 out]
        n363 = case shown="0, Default" "MCL Mode" {
          tunnel: w677 -> [_ w680 w727]
          frame 0, Default {
            # "manual positioning"
          }
          frame 1 {
            # "sinusoidal wave"
            n364 = node-c288() -> (w682:T25)  [unwired: 4 out]
            n365 = timed-loop "Oscillate MCL mirror" {
              timing: w682 -> [_]
              timing-out: [_] -> w681
              tunnel: w680 -> [w721]
              i -> [w720]
              stop <- w683 stop-if-true
              n366 = node-c288() -> (w719:i64)  [unwired: 1 out]
              n367 = Multiply(x="AO1", y=32767.0) -> (x*y=w715:dbl)
              n368 = Multiply(x="AO2", y=32767.0) -> (x*y=w710:dbl)
              n369 = Divide(x=w715, y=10.0) -> (x/y=w716:dbl)
              n370 = Divide(x=w710, y=10.0) -> (x/y=w711:dbl)
              n371 = To Word Integer(number=w716) -> (16bit integer=w708:i16)
              n372 = To Word Integer(number=w711) -> (16bit integer=w707:i16)
              n373 = Divide(x=w719, y=i64 1000) -> (x/y=w690:dbl)
              n374 = Multiply(x=w690, y=w720) -> (x*y=w701:dbl)
              n375 = Multiply(x="Osc. freq. (Hz) 2", y=6.283185307179586) -> (x*y=w702:dbl)
              n376 = Multiply(x=w702, y=w701) -> (x*y=w700:dbl)
              n377 = Sine(x=w700) -> (sin(x)=w699:dbl)
              n378 = Multiply(x=w699, y="Osc. amp. (V)") -> (x*y=w697:dbl)
              n379 = Add(x=w697, y="Osc. center (V)") -> (x+y=w695:dbl)
              n380 = Divide(x=w695, y=10.0) -> (x/y=w693:dbl)
              n381 = Multiply(x=w693, y=32767.0) -> (x*y=w688:dbl)
              n382 = Select(t=w688, s="Scan axis", f=w708) -> (s? t:f=w706:dbl)
              n383 = Select(t=w707, s="Scan axis", f=w688) -> (s? t:f=w705:dbl)
              n384 = local read "MCL Mode"() -> (w687:u16)
              n385 = Not Equal?(x=w687, y=u16 1) -> (x != y?=w684:bool)
              n386 = local read "Stop All"() -> (w685:bool)
              n387 = xnode "Read/Write Control"("FPGA VI Reference In"=w721, "AO1 (Y)"=w706, "AO2 (X)"=w705) -> ()  [unwired: 1 in, 2 out]
              n388 = Compound Arithmetic op=OR(w685, w684) -> (w683:bool)
              n389 = node-c288() -> ()  [unwired: 2 out]
            }
            n390 = node-c288(w681) -> ()  [unwired: 1 out]
          }
          frame 2 {
            # "linear scan"
            n391 = case shown="True" "Start Scan" {
              tunnel: w727 -> [_ w739]
              frame False {
              }
              frame True {
                n392 = Subtract(x="End (V)", y="Begin (V)") -> (x-y=w735:dbl)
                n393 = Decrement(x="N Points") -> (x-1=w734:dbl)
                n394 = Divide(x=w735, y=w734) -> (x/y=w732:dbl)
                n395 = for {
                  N: "N Points" -> [_]
                  tunnel: "Begin (V)" -> [w752]
                  tunnel: w739 -> [w744]
                  tunnel: [w743] -> w738 mode=indexing
                  tunnel: w732 -> [w742]
                  tunnel: [w740] -> w731 mode=indexing
                  i -> [w751]
                  n396 = Multiply(x=w742, y=w751) -> (x*y=w750:dbl)
                  n397 = Add(x=w752, y=w750) -> (x+y=w747:dbl)
                  n398 = local read "Scan axis"() -> (w741:bool)
                  n399 = local read "AO1"() -> (w749:dbl)
                  n400 = local read "AO2"() -> (w748:dbl)
                  n401 = Select(t=w747, s=w741, f=w749) -> (s? t:f=w746:dbl)
                  n402 = Select(t=w748, s=w741, f=w747) -> (s? t:f=w745:dbl)
                  n403 = flat-sequence {
                    tunnel: w746 -> [w756]
                    tunnel: w745 -> [w755]
                    tunnel: w744 -> [w753]
                    tunnel: [w766] -> w743
                    tunnel: [w765] -> w740
                    frame #0 {
                      w759 = 10.0 ("y")
                      w754 = 32767.0 ("y")
                      n404 = Multiply(x=w756, y=w754) -> (x*y=w762:dbl)
                      n405 = Multiply(x=w755, y=w754) -> (x*y=w760:dbl)
                      n406 = Divide(x=w762, y=w759) -> (x/y=w763:dbl)
                      n407 = Divide(x=w760, y=w759) -> (x/y=w761:dbl)
                      n408 = To Word Integer(number=w763) -> (16bit integer=w757:i16)
                      n409 = To Word Integer(number=w761) -> (16bit integer=w758:i16)
                      n410 = xnode "Read/Write Control"("FPGA VI Reference In"=w753, "AO1 (Y)"=w757, "AO2 (X)"=w758) -> ()  [unwired: 1 in, 2 out]
                    }
                    frame #1 {
                      n411 = Wait (ms)(milliseconds to wait="DAQ Delay (ms)") -> ()  [unwired: 1 out]
                    }
                    frame #2 {
                      n412 = local read "Slow mean"() -> (w766:dbl)
                      n413 = local read "Sigma"() -> (w765:dbl)
                    }
                  }
                }
                n414 = Bundle("Begin (V)"="Begin (V)", w732, w738) -> (→"MCL Scan":cluster{"Begin (V)":dbl, dbl, dbl[]})  [unwired: 1 out]
                n415 = Bundle("Begin (V)"="Begin (V)", w732, w731) -> (→"MCL Scan 2":cluster{"Begin (V)":dbl, dbl, dbl[]})  [unwired: 1 out]
              }
            }
          }
        }
        n416 = local read "Stop All"() -> (w676:bool)
        n417 = node-c288() -> ()  [unwired: 2 out]
      }
      n418 = node-c288(w673) -> ()  [unwired: 1 out]
    }
    frame Disabled {
    }
  }
  n419 = node-c288(2 ("Processor")) -> (w52:T25)  [unwired: 3 in]
  n420 = timed-loop "Control parameters (event loop)" {
    tunnel: w59 -> [w772]
    shift-right: [w771] -> _
    shift-left: errorcluster {"status"=FALSE, "code"=0, "source"=""} ("error out") -> [w770]
    tunnel: [w769] -> w72
    timing: w52 -> [_]
    timing-out: [_] -> w51
    stop <- w769 stop-if-true
    n421 = node-c288() -> ()  [unwired: 1 in, 1 out]
    n422 = event shown="[33] \"Scan steps (MCL)\", \"Number of scans (MCL)\", \"Scan Range (V) (of steps)\", \"2D or 1D Scan\", \"N APD Samp/step\", \"Fast Scan Dir\", \"Continuous MCL Scanning\", \"Scan lines (y)\": Value Change" {
      selector: _ -> [_ _ _ _ _ _ _ _ _ _ _ _ _ _ _ _ _ _ _ _ _ _ _ _ _ _ _ _ _ _ _ _ _ _ _ _ _ _ _ _ _ _ _ _ _ _ _ _ _ _ _ _ _ _ _ _ _ _ _ _ _]
      dyn-events: _ -> [_ _ _ _ _ _ _ _ _ _ _ _ _ _ _ _ _ _ _ _ _ _ _ _ _ _ _ _ _ _ _ _ _ _ _ _ _ _ _ _ _ _ _ _ _ _ _ _ _ _ _ _ _ _ _ _ _ _ _ _ _]
      timeout: _ -> [_ _ _ _ _ _ _ _ _ _ _ _ _ _ _ _ _ _ _ _ _ _ _ _ _ _ _ _ _ _ _ _ _ _ _ _ _ _ _ _ _ _ _ _ _ _ _ _ _ _ _ _ _ _ _ _ _ _ _ _ _]
      tunnel: w772 -> [w813 _ _ _ w850 _ w868 w874 _ _ _ _ w951 _ _ w995 w1001 w1005 w1010 w1046 w1064 w1071 w1089 w1100 w1111 w1122 w1133 w1144 w1162 w1168 w1262 _ w1274 w1312 _ w1385 w1389 w1400 w1405 w1429 _ w1437 _ _ _ _ _ w1573 _ w1590 w1605 w1631 w1634 w1657 w1717 _ w1734 w1737 _ _ _]
      tunnel: [w812 _ _ _ w840 _ _ w873 _ _ w916 _ w931 _ _ w994 w997 w1004 w1007 w1045 w1062 w1070 w1083 w1094 w1105 w1116 w1127 w1138 w1160 w1167 w1260 _ w1272 w1310 _ w1383 w1387 w1390 w1403 w1427 _ w1435 _ _ _ _ _ w1571 _ _ _ _ _ _ _ _ _ _ _ _ _] -> w771
      tunnel: w770 -> [w811 _ _ _ w849 _ _ w872 _ _ w916 _ w950 _ _ w993 w996 w1003 w1006 w1044 w1063 w1069 w1088 w1099 w1110 w1121 w1132 w1143 w1161 w1166 w1261 _ w1273 w1311 _ w1384 w1388 w1399 w1404 w1428 _ w1436 _ _ _ _ _ w1572 _ w1589 w1604 w1630 w1633 w1658 w1716 _ w1733 _ _ _ _]
      tunnel: [_ _ _ _ _ _ _ _ _ _ w915 _ _ _ _ _ _ _ _ _ _ _ _ _ _ _ _ _ _ _ _ _ _ _ _ _ _ _ _ _ _ _ _ _ _ _ _ _ _ _ _ _ _ _ _ _ _ _ _ _ _] -> w769
      tunnel: [_ _ _ _ _ _ _ _ "Round T1 X" _ _ _ _ _ _ _ _ _ _ _ _ _ _ _ _ _ _ _ _ _ _ _ _ _ _ _ _ _ _ _ _ _ _ _ _ _ _ _ _ _ _ _ _ _ _ _ _ _ _ _ _] -> _
      tunnel: [_ _ _ "Adjust Scale\nto Mean" _ _ _ _ _ _ _ _ _ _ _ _ _ _ _ _ _ _ _ _ _ _ _ _ _ _ _ _ _ _ _ _ _ _ _ _ _ _ _ _ _ _ _ _ _ _ _ _ _ _ "Set SP to Reading" _ _ _ _ _ _] -> _
      tunnel: [_ _ _ _ _ _ _ _ _ "Round T2 X" _ "Delayed Interlace Start" _ _ _ _ _ _ _ _ _ _ _ _ _ _ _ _ _ _ _ _ _ _ _ _ _ _ _ _ _ _ _ _ _ _ _ _ _ _ _ _ _ _ _ _ _ _ _ _ _] -> _
      event "AI Count (ticks)", "Sets to FIFO (Traps)", "Save ave N", "FPGA Ave.", "# Samples/channel", "N sets to save": Value Change {
        # "So that if 'Save ave N' is updated, the AOD scanning code updates too."
        n423 = event-data() -> ()  [unwired: 6 out]
        n424 = local read "AI Count (ticks)"() -> (w794:u32)
        n425 = Unbundle By Name("Sets to FIFO (Traps)") -> ("Set 1"=w777:bool, "Set 2"=w776:bool, "Set 3"=w775:bool)
        n426 = Boolean To (0,1)(Boolean="Sets to FIFO (Traps)") -> (0, 1=w803:cluster{"Set 1":i16, "Set 2":i16, "Set 3":i16})
        n427 = xnode "Read/Write Control"("FPGA VI Reference In"=w813, "error in"=w811, "ai count"=w794, "Set 1"=w777, "Set 2"=w776, "Set 3"=w775, "N of AI1 Int Acq Sets"="N Acq Sets (Traps + Fl.)") -> ("error out"=w812:errorcluster)  [unwired: 1 out]
        n428 = Cluster To Array(cluster=w803) -> (array=w802:i16[])
        n429 = To Unsigned Long Integer(number=w802) -> (unsigned 32bit integer=w783:u32[])
        n430 = local read "Scan steps (AOD)"() -> (w804:u64)
        n431 = Multiply(x=w794, y="N Acq Sets (Traps + Fl.)") -> (x*y=w792:u32)
        n432 = Divide(x=40000000.0, y=w794) -> (x/y=w786:dbl)
        "AI rate (Hz)" <- w786
        "Ave. Rate (Hz)" <- w786
        n433 = Add Array Elements(numeric array=w783) -> (sum=w795:u32)
        "Trap Sets" <- w795
        n434 = Reciprocal(x=w786) -> (1/x=→"Ave. Period (s)":dbl)
        n435 = property on="Scan steps (AOD)" class="DigNum (strict)"("Val(Sgnl)"=w804) -> ()  [unwired: 2 in, 2 out]
        n436 = Divide(x=w786, y="N Acq Sets (Traps + Fl.)") -> (x/y=w808:dbl)
        "Data Rate (Hz)" <- w808
        n437 = Reciprocal(x=w808) -> (1/x=→"Data Period (s)":dbl)
        n438 = local read "Save ave N"() -> (w807:dbl)
        n439 = Divide(x=w808, y=w807) -> (x/y=w806:dbl)
        "Save Data Rate (Hz)" <- w806
        n440 = Reciprocal(x=w806) -> (1/x=→"Save Data Period (s)":dbl)
        n441 = Multiply(x=w792, y="# Samples/trap") -> (x*y=w790:u32)
        "Counts/DMA" <- w790
        n442 = property on="Trap Disp. Downsample" class="DigNum (strict)"("Maximum"="# Samples/trap") -> ()  [unwired: 2 in, 2 out]
        n443 = Multiply(x=w795, y="# Samples/trap") -> (x*y=w784:u32)
        "# Samples/channel" <- w784
        n444 = Multiply(x=w784, y=u32 8) -> (x*y=→"Trap AI Elements/DMA read":u32)
        n445 = local read "APD Int. Count"() -> (w791:u32)
        n446 = Multiply(x=w784, y=u32 3) -> (x*y=→"Trap Pos Elements/DMA read":u32)
        n447 = Divide(x=w790, y=w791) -> (x/y=w781:dbl)
        "APD Samples/FIFO Acq." <- w781
        n448 = Divide(x=w790, y=40000000.0) -> (x/y=w788:dbl)
        "DMA Update Period (s)" <- w788
        n449 = Multiply(x=2.0, y=w781) -> (x*y=→"APD Elements/DMA read":dbl)
        n450 = property on="APD Disp. Downsample" class="DigNum (strict)"("Maximum"=w781) -> ()  [unwired: 2 in, 2 out]
        n451 = local read "N sets to save"() -> (w800:u32)
        n452 = Multiply(x=w788, y=w800) -> (x*y=→"Total Time (s)":dbl)
        "FPGA Averaging" <- FALSE ("FPGA Averaging")
      }
      event "Rescale on Mean": Value Change {
        n453 = event-data() -> ()  [unwired: 7 out]
        n454 = And(x=FALSE, y="Rescale on Mean") -> (x .and. y?=w815:bool)
        n455 = local write "Rescale on Mean"(w815) -> ()
        n456 = local read "Bead Mean (nm)"() -> (w820:dbl)
        n457 = Add(x="Amplitude (nm)", y=w820) -> (x+y=w818:dbl)
        n458 = Subtract(x=w820, y="Amplitude (nm)") -> (x-y=w817:dbl)
        n459 = property on="Bead Separation" class="WFChart (strict)"("YScale.Minimum"=w817) -> ()  [unwired: 2 in, 2 out]
        n460 = property on="Bead Separation" class="WFChart (strict)"("YScale.Maximum"=w818) -> ()  [unwired: 2 in, 2 out]
      }
      event "Detector Type": Value Change {
        n461 = event-data() -> ()  [unwired: 7 out]
        n462 = local read "AI labels"() -> (w821:string[])
        n463 = property on="High Res. Display" class="Ring (strict)"("Strings []"=w821) -> ()  [unwired: 2 in, 2 out]
        n464 = Build Array (concatenate)(w821, "none") -> (w822:string[])
        n465 = property on="FFT 1 Choice 1" class="Ring (strict)"("Strings []"=w822) -> ()  [unwired: 2 in, 2 out]
        n466 = property on="FFT 1 Choice 2" class="Ring (strict)"("Strings []"=w822) -> ()  [unwired: 2 in, 2 out]
        n467 = property on="FFT 2 Choice 1" class="Ring (strict)"("Strings []"=w822) -> ()  [unwired: 2 in, 2 out]
        n468 = property on="FFT 2 Choice 2" class="Ring (strict)"("Strings []"=w822) -> ()  [unwired: 2 in, 2 out]
        n469 = Bundle("APD 1", "APD 2") -> (w825:cluster{string, string})  [unwired: 1 out]
        n470 = Cluster To Array(cluster=w825) -> (array=w823:string[])
        n471 = Build Array (concatenate)(w823, w822) -> (w827:string[])
        n472 = Array Size(array=w827) -> (size(s)=w828:i32)
        n473 = property on="Signals to Plot" class="LstBox (strict)"("Item Names"=w827) -> ()  [unwired: 2 in, 2 out]
        n474 = property on="Signals to Plot" class="LstBox (strict)"("Number of Rows"=w828) -> ()  [unwired: 2 in, 2 out]
        n475 = property on="All Signals" class="WFChart (strict)"("LegNumRows"=w828) -> ()  [unwired: 2 in, 2 out]
      }
      event "Adjust Scale\nto Mean": Value Change {
        n476 = event-data() -> ()  [unwired: 7 out]
        n477 = local read "APD 1 Rate (Hz)"() -> (w837:dbl)
        n478 = Multiply(x=1000.0, y="Above (kHz)") -> (x*y=w835:dbl)
        n479 = Multiply(x=1000.0, y="Below (kHz)") -> (x*y=w833:dbl)
        n480 = Add(x=w835, y=w837) -> (x+y=w830:dbl)
        n481 = Subtract(x=w837, y=w833) -> (x-y=w831:dbl)
        n482 = property on="APD Chart" class="WFChart (strict)"("YScale.Minimum"=w831) -> ()  [unwired: 2 in, 2 out]
